vi "fpga.vi"() -> ()   [LabVIEW 2015]
uses:
  <vilib>/rvi/eio/common/nirviEmuTemplateMethod_errors.vi
  <vilib>/eio/EIONode/EIONode.xnode
panel:
  out "Reset":bool
  out "Set":bool
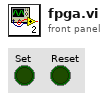
[diagram p1: front panel]
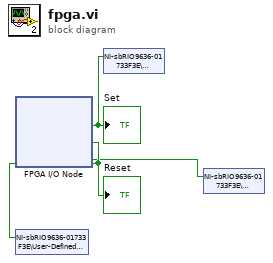
[diagram p0: block diagram]
diagram:
  n1 = xnode "FPGA I/O Node"() -> ("DIO12"=w3:bool, "DIO16"=w2:bool, "DIO15"=w1:bool)  [unwired: 3 in, 3 out]
  "Set" <- w3
  "Reset" <- w2
  n2 = shared-variable "NI-sbRIO9636-01733F3E\\User-Defined Variables\\Reset"(w2) -> ()  [unwired: 1 in, 1 out]
  n3 = shared-variable "NI-sbRIO9636-01733F3E\\User-Defined Variables\\Set"(w3) -> ()  [unwired: 1 in, 1 out]
  n4 = shared-variable "NI-sbRIO9636-01733F3E\\User-Defined Variables\\On"(w1) -> ()  [unwired: 1 in, 1 out]
